vi "PH_Sixpack.PC SetPeakCurrent.vi"(0 "i ref in":refnum<vi>, 1 "Axis":i32=-1, 2 "Imax (50%)":T1=50.0 min=0.0 max=100.0, 3 "To set?":bool, 5 "error in":errorcluster) -> (14 "i ref out":refnum<vi>, 16 "ok?":bool, 19 "error out":errorcluster)   [LabVIEW 2014, in "PH_Sixpack.lvlib"]
doc: "This VI stores information to own attributes."
uses:
  PH_Sixpack.lvlib
  instr.lib/Sixpack/PackDLL/PeakCurrent.ctl
  instr.lib/Sixpack/Sixpack - Driver.lvlib
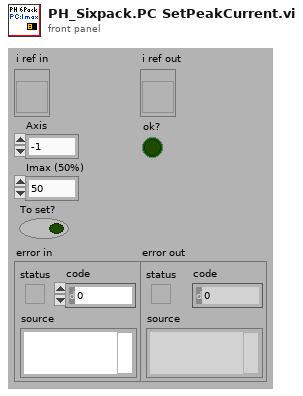
[diagram p1: front panel]
types:
  T1 = typedef "Sixpack - Driver.lvlib/PeakCurrent.ctl" = dbl
  T2 = typedef "PH_Sixpack.lvlib/PH_Sixpack.i attribute.ctl" = cluster{"Information":cluster{"SixPack ID(0)":u16, "BaudRate(19200)":u16, "COM Port":enum32{"COM1", "COM2", "COM3", "COM4", "COM5", "COM6", "COM7", "COM8", "COM9"}, "HANDLE":i32}, "Serial Number":dbl, "Firmwareversion":dbl, "Axes":T3[], "Status":T14, "Axis to do a RefSearch":i32, "GUI Refs":cluster{"Information":refnum<vi>, "Serial Number":refnum<vi>, "Firmwareversion":refnum<vi>, "Status":refnum<vi>, "Axis to do a RefSearch":refnum<vi>, "Axes Configuration (Sixpack)":refnum<vi>, "Inputs":refnum<vi>, "PeriodicInterval [ms]":refnum<vi>}, "Constructor finished":bool, "Ignore Error":bool}
  T3 = typedef "PH_Sixpack.lvlib/PH_Sixpack.Axis Cluster.ctl" = cluster{"Config":T4, "To set?":cluster{"VmaxAmax":bool, "I max":bool, "VStartVminDivi":bool, "Ref Search Parameter":bool, "Stopswitch Limits":bool, "Axis Parameter":bool, "I Control":bool}}
  T4 = typedef "PH_Sixpack.lvlib/PH_Sixpack.Axis Configuration.ctl" = cluster{"VmaxAmax":T5, "I max (50%)":T1, "VStartVminDivi":T6, "Ref Search Parameter":T7, "Stopswitch Limits":T8, "Axis Parameter":T9, "I Control":T12}
  T5 = typedef "Sixpack - Driver.lvlib/VmaxAmax.ctl" = cluster{"VMax(511)":u16, "AMax(128)":u16}
  T6 = typedef "Sixpack - Driver.lvlib/VStartVmin.ctl" = cluster{"VStart(5)":u16, "Vmin(4)":u16, "Div i (2)":enum8{"0", "1", "2", "3"}}
  T7 = typedef "Sixpack - Driver.lvlib/Ref Search Parameter.ctl" = cluster{"VRefMax(100)":u16, "DebouncingTime (22ms)":u8}
  T8 = typedef "Sixpack - Driver.lvlib/Stopswitch Limits.ctl" = cluster{"MinLeft(0)":u16, "MaxRight(1023)":u16}
  T9 = typedef "Sixpack - Driver.lvlib/Motor Parameter.ctl" = cluster{"Poslimit (6400)":u32, "P5 Bits":T10, "P6 Bits":T11}
  T10 = typedef "Sixpack - Driver.lvlib/MotorParameter_P5.ctl" = cluster{"MT_PI":bool, "MT_ROTARY":bool, "MT_AUTONULLCMD":bool, "MT_TESTNULL":bool, "MT_NULLLEFT":bool, "MT_NULLCENTRE":bool, "MT_STOPNULL":bool, "MT_FILTERSWITCH":bool}
  T11 = typedef "Sixpack - Driver.lvlib/MotorParameter_P6.ctl" = cluster{"MT_OPTIMIZEWAY":bool, "MT_FASTREF":bool, "MT_MECHREF":bool, "MT_DELAYTESTNULL":bool, "MT_STOPSOFT":bool, "MT_STOPNOREF":bool, "MT_NULLPOSITIVE":bool, "MUT_STOPFULSTEPS":bool}
  T12 = typedef "Sixpack - Driver.lvlib/Current Control.ctl" = cluster{"PowerDownDelay (500)":u16, "PowerDown (0%)":T13, "Standing (50%)":T13, "Running (75%)":T13, "Accelerating (100%)":T13}
  T13 = typedef "Sixpack - Driver.lvlib/Current.ctl" = enum8{"100%", "75%", "50%", "38%", "25%", "19%", "13%", "9%", "0%"}
  T14 = typedef "PH_Sixpack.lvlib/PH_Sixpack.Status.ctl" = enum32{"None", "Init", "Configure", "configured", "Close", "closed"}
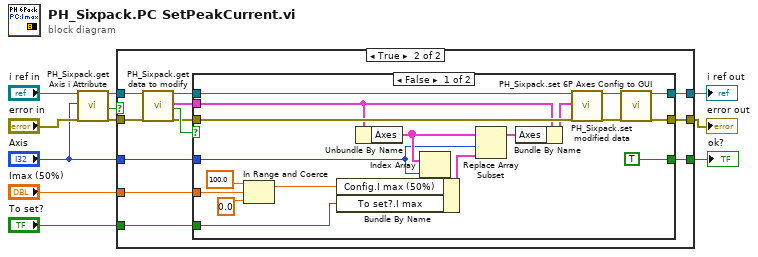
[diagram p0: block diagram]
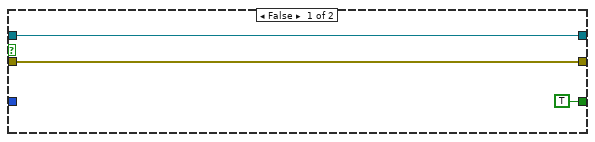
[diagram p2: hidden frame]
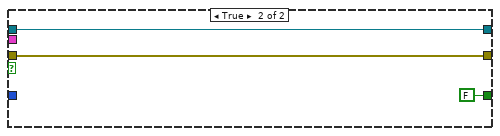
[diagram p3: hidden frame]
diagram:
  n1 = call "PH_Sixpack.get Axis i Attribute.vi"("VI in"="i ref in", "Axis"="Axis", "error in"="error in") -> ("VI out"=w6:refnum<vi>, "Axis found?"=w3:bool, "error out"=w8:errorcluster)  [unwired: 10 in, 4 out]
  n2 = case shown="True" w3 {
    tunnel: [w13 w24] -> w10
    tunnel: [w14 w22] -> w9
    tunnel: w8 -> [w13 w20]
    tunnel: w6 -> [w14 w19]
    tunnel: "Axis" -> [_ w18]
    tunnel: "Imax (50%)" -> [_ w17]
    tunnel: "To set?" -> [_ w16]
    tunnel: [TRUE w15] -> w1
    frame False {
    }
    frame True {
      n3 = call "PH_Sixpack.get data to modify.vi"("i ref in"=w19, "error in (no error)"=w20) -> ("i ref out"=w23:refnum<vi>, "i attribute"=w21:T2, "timed out"=w26:bool, "error out"=w25:errorcluster)  [unwired: 14 in]
      n4 = case shown="False" w26 {
        tunnel: [w30 w48] -> w24
        tunnel: w25 -> [w43 w48]
        tunnel: [w28 w47] -> w22
        tunnel: w23 -> [w44 w47]
        tunnel: w21 -> [w42 _]
        tunnel: w18 -> [w33 _]
        tunnel: w17 -> [w40 _]
        tunnel: w16 -> [w31 _]
        tunnel: [TRUE FALSE] -> w15
        frame False {
          n5 = In Range and Coerce(upper limit=100.0, x=w40, lower limit=0.0) -> (coerced(x)=w34:T1)  [unwired: 1 out]
          n6 = Unbundle By Name(w42) -> ("Axes"=w45:T3[])
          n7 = Index Array(array=w45, index=w33) -> (element=w35:T3)
          n8 = Bundle By Name(cluster=w35, "Config.I max (50%)"=w34, "To set?.I max"=w31) -> (w37:T3)
          n9 = Replace Array Subset(array=w45, new element=w37, index=w33) -> (w36:T3[])
          n10 = Bundle By Name(cluster=w42, "Axes"=w36) -> (w41:T2)
          n11 = call "PH_Sixpack.set modified data.vi"("i ref in"=w44, "i attribute"=w41, "error in (no error)"=w43) -> ("i ref out"=w29:refnum<vi>, "error out"=w32:errorcluster)  [unwired: 15 in]
          n12 = call "PH_Sixpack.set 6P Axes Config to GUI.vi"("VI in"=w29, "error in (no error)"=w32) -> ("VI out"=w28:refnum<vi>, "error out"=w30:errorcluster)  [unwired: 16 in]
        }
        frame True {
        }
      }
    }
  }
  "error out" <- w10
  "i ref out" <- w9
  "ok?" <- w1
